vi "SVI_Calculate_checksum.vi"(1 "Message":string) -> (0 "Calculated checksum":string)   [LabVIEW 2014]
panel:
  out "Split array":string[](array[string])
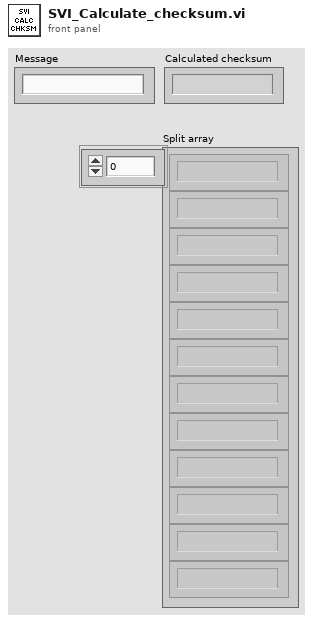
[diagram p1: front panel]
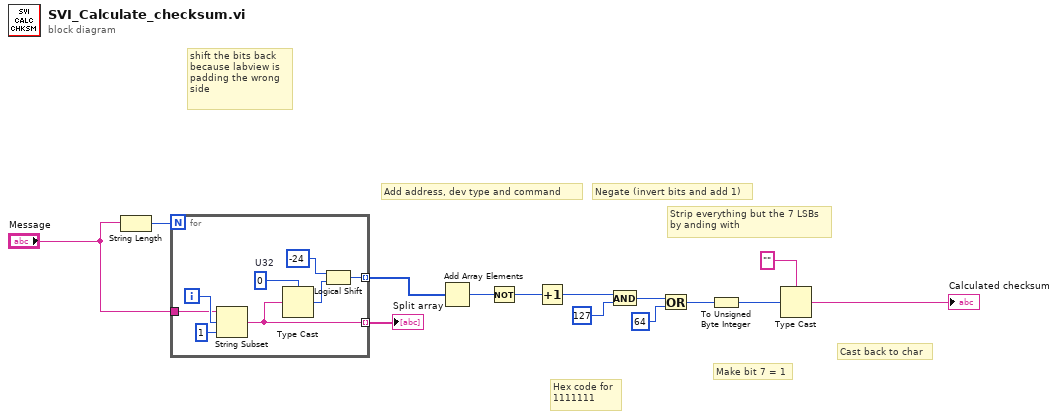
[diagram p0: block diagram]
diagram:
  # "shift the bits back\nbecause labview is \npadding the wrong\nside"
  # "Cast back to char"
  # "Hex code for\n1111111"
  # "Make bit 7 = 1"
  # "Strip everything but the 7 LSBs\nby anding with"
  # "Negate (invert bits and add 1)"
  # "Add address, dev type and command"
  n1 = String Length(string="Message") -> (length=w9:i32)
  n2 = for {
    N: w9 -> [_]
    tunnel: "Message" -> [w21]
    tunnel: [w15] -> w8 mode=indexing
    tunnel: [w19] -> w10 mode=indexing
    i -> [w22]
    w20 = u32 0  # U32
    n3 = String Subset(string=w21, offset (0)=w22, length (rest)=1 ("length (rest)")) -> (substring=w19:string)
    n4 = Type Cast(type=w20, x=w19) -> (*(type *) &x=w17:u32)
    n5 = Logical Shift(y=i16 -24, x=w17) -> (x << y=w15:u32)
  }
  "Split array" <- w10
  n6 = Add Array Elements(numeric array=w8) -> (sum=w7:u32)
  n7 = Not(x=w7) -> (.not. x?=w11:u32)
  n8 = Increment(x=w11) -> (x+1=w13:u32)
  n9 = And(x=w13, y=u32 127) -> (x .and. y?=w12:u32)
  n10 = Or(x=w12, y=u32 64) -> (x .or. y?=w4:u32)
  n11 = To Unsigned Byte Integer(number=w4) -> (unsigned 8bit integer=w1:u8)
  n12 = Type Cast(type="", x=w1) -> (*(type *) &x=→"Calculated checksum":string)
